vi "上下巡检模块.vi"(2 "巡检时间间隔":dbl, 3 "连接ID":refnum<k5>) -> ()   [LabVIEW 2015]
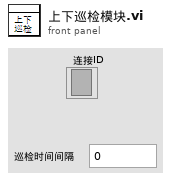
[diagram p1: front panel]
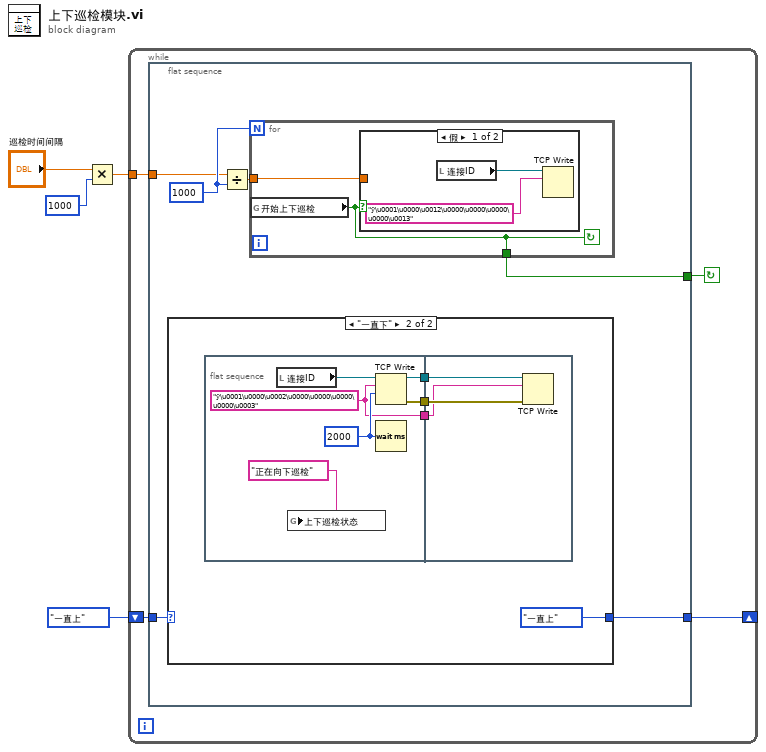
[diagram p0: block diagram]
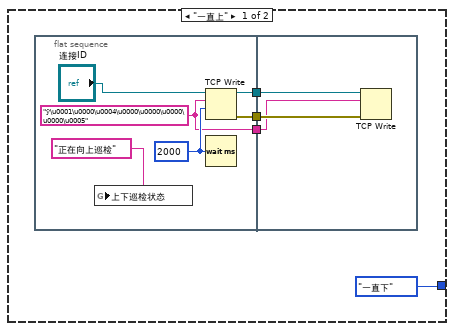
[diagram p2: hidden frame]
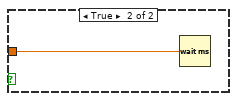
[diagram p3: hidden frame]
diagram:
  n1 = Multiply(x="巡检时间间隔", y=1000) -> (x*y=w2:dbl)
  n2 = while {
    tunnel: w2 -> [w8]
    shift-right: [w6] -> _
    shift-left: enum16{"一直上", "一直下"}."一直上" -> [w7]
    stop <- w5 continue-if-true
    n3 = flat-sequence {
      tunnel: w8 -> [w12]
      tunnel: w7 -> [w11]
      tunnel: [w10] -> w6
      tunnel: [w9] -> w5
      frame #0 {
        w13 = 1000
        n4 = case shown="\"一直下\"" w11 {
          tunnel: [enum16{"一直上", "一直下"}."一直下" enum16{"一直上", "一直下"}."一直上"] -> w10
          frame "一直上" {
            n5 = flat-sequence {
              tunnel: [w23] -> w18
              tunnel: [w22] -> w17
              tunnel: [w21] -> w16
              tunnel: w18 -> [w27]
              tunnel: w17 -> [w26]
              tunnel: w16 -> [w25]
              frame #0 {
                w24 = 2000
                w21 = "ÿ\u0001\u0000\u0004\u0000\u0000\u0000\u0000\u0005"
                n6 = global write "导轨控制全局.vi" "上下巡检状态"("正在向上巡检") -> ()
                n7 = TCP Write(connection ID="连接ID", data in=w21, 9:w24) -> (connection ID out=w22:refnum<k5>, error out=w23:errorcluster)  [unwired: 1 in, 1 out]
                n8 = Wait (ms)(milliseconds to wait=w24) -> ()  [unwired: 1 out]
              }
              frame #1 {
                n9 = TCP Write(connection ID=w26, data in=w25, error in (no error)=w27) -> ()  [unwired: 1 in, 3 out]
              }
            }
          }
          frame "一直下" {
            n10 = flat-sequence {
              tunnel: [w35] -> w31
              tunnel: [w34] -> w30
              tunnel: [w33] -> w28
              tunnel: w31 -> [w40]
              tunnel: w30 -> [w39]
              tunnel: w28 -> [w38]
              frame #0 {
                w37 = 2000
                w33 = "ÿ\u0001\u0000\u0002\u0000\u0000\u0000\u0000\u0003"
                n11 = local read "连接ID"() -> (w36:refnum<k5>)
                n12 = global write "导轨控制全局.vi" "上下巡检状态"("正在向下巡检") -> ()
                n13 = TCP Write(connection ID=w36, data in=w33, 9:w37) -> (connection ID out=w34:refnum<k5>, error out=w35:errorcluster)  [unwired: 1 in, 1 out]
                n14 = Wait (ms)(milliseconds to wait=w37) -> ()  [unwired: 1 out]
              }
              frame #1 {
                n15 = TCP Write(connection ID=w39, data in=w38, error in (no error)=w40) -> ()  [unwired: 1 in, 3 out]
              }
            }
          }
        }
        n16 = Divide(x=w12, y=w13) -> (x/y=w14:dbl)
        n17 = for {
          N: w13 -> [_]
          tunnel: w14 -> [w42]
          tunnel: [w41] -> w9
          stop <- w41 continue-if-true
          n18 = global read "导轨控制全局.vi" "开始上下巡检"() -> (w41:bool)
          n19 = case shown="假" w41 {
            tunnel: w42 -> [_ w45]
            frame False {
              n20 = local read "连接ID"() -> (w44:refnum<k5>)
              n21 = TCP Write(connection ID=w44, data in="ÿ\u0001\u0000\u0012\u0000\u0000\u0000\u0000\u0013") -> ()  [unwired: 2 in, 3 out]
            }
            frame True {
              n22 = Wait (ms)(milliseconds to wait=w45) -> ()  [unwired: 1 out]
            }
          }
        }
      }
    }
  }
